vi "Tosca-Randomize Parameter Family.vi"(0 "Family in":T1, 7 "Mode":T5, 11 "N":i32) -> (4 "Family thru":T1, 8 "SCL":T6[](array[typedef]))   [LabVIEW 2020]
uses:
  Typedefs/Tosca-Parameter Family.ctl
  Typedefs/Tosca-Parameter Table Element.ctl
  Typedefs/Tosca-Parameter Dimension.ctl
  Typedefs/Tosca-Family Order.ctl
  Typedefs/Tosca-SCL Element.ctl
  Typedefs/Tosca-Schedule Mode.ctl
  Typedefs/Tosca-Event Type.ctl
  Typedefs/Tosca-SCL Variable.ctl
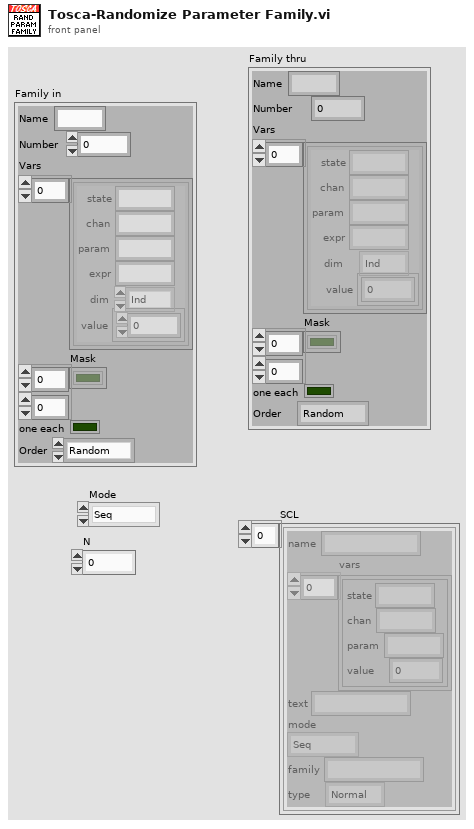
[diagram p1: front panel]
types:
  T1 = typedef "Tosca-Parameter Family.ctl" = cluster{"Name":string, "Number":i32, "Vars":T2[], "Mask":bool[][], "one each":bool, "Order":T4}
  T2 = typedef "Tosca-Parameter Table Element.ctl" = cluster{"state":string, "chan":string, "param":string, "expr":string, "dim":T3, "value":dbl[]}
  T3 = typedef "Tosca-Parameter Dimension.ctl" = enum16{"Ind", "X", "Y"}
  T4 = typedef "Tosca-Family Order.ctl" = enum16{"Random", "Sequential"}
  T5 = typedef "Tosca-Schedule Mode.ctl" = enum16{"Seq", "CS+/CS-", "Adapt"}
  T6 = typedef "Tosca-SCL Element.ctl" = cluster{"name":string, "vars":cluster{"state":string, "chan":string, "param":string, "value":dbl}[], "text":string, "mode":T5, "family":string, "type":T7}
  T7 = typedef "Tosca-Event Type.ctl" = enum16{"Normal", "CS+", "CS-"}
  T8 = typedef "Tosca-SCL Variable.ctl" = cluster{"state":string, "chan":string, "param":string, "value":dbl}
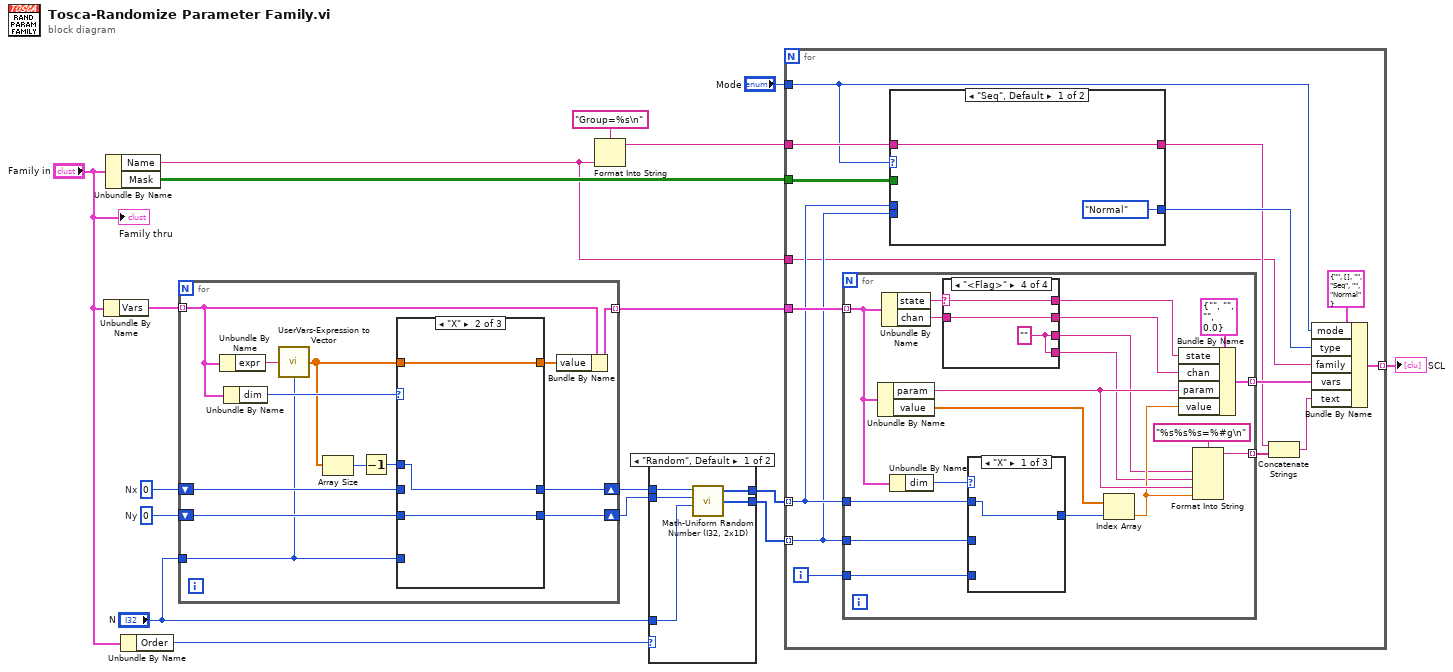
[diagram p0: block diagram]
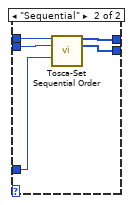
[diagram p2: hidden frame]
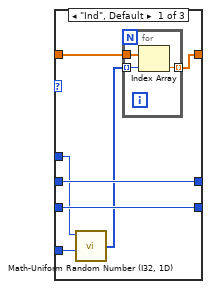
[diagram p3: hidden frame]
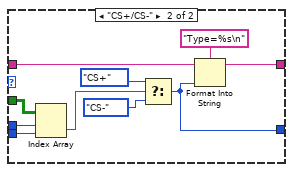
[diagram p5: hidden frame]
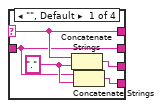
[diagram p6: hidden frame]
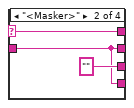
[diagram p7: hidden frame]
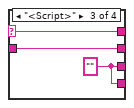
[diagram p8: hidden frame]
diagram:
  w15 = 0  # Ny
  w16 = 0  # Nx
  n1 = Unbundle By Name("Family in") -> ("Vars"=w17:T2[])
  n2 = Unbundle By Name("Family in") -> ("Name"=w8:string, "Mask"=w11:bool[][])
  n3 = Unbundle By Name("Family in") -> ("Order"=w1:T4)
  n4 = for {
    tunnel: w17 -> [w23] mode=indexing
    shift-right: [w27] -> w5
    shift-left: w16 -> [w26]
    shift-right: [w25] -> w4
    shift-left: w15 -> [w24]
    tunnel: [w22] -> w14 mode=indexing
    tunnel: "N" -> [w18]
    n5 = Unbundle By Name(w23) -> ("expr"=w30:string)
    n6 = Unbundle By Name(w23) -> ("dim"=w29:T3)
    n7 = call "UserVars-Expression to Vector.vi"("Expr"=w30, "Nrand"=w18) -> ("Values"=w20:dbl[])  [unwired: 12 in, 1 out]
    n8 = Array Size(array=w20) -> (size(s)=w28:i32)
    n9 = Decrement(x=w28) -> (x-1=w19:i32)
    n10 = case shown="\"X\"" w29 {
      tunnel: w19 -> [w35 w42 w46]
      tunnel: [w37 w42 w45] -> w27
      tunnel: w26 -> [w37 _ w45]
      tunnel: [w36 w43 w46] -> w25
      tunnel: w24 -> [w36 w43 _]
      tunnel: w18 -> [w34 _ _]
      tunnel: [w32 w41 w44] -> w21
      tunnel: w20 -> [w33 w41 w44]
      frame "Ind", Default {
        n11 = call "Math-Uniform Random Number (I32, 1D).vi"("N"=w34, "Ymax"=w35) -> ("Random Ints"=w31:i32[])  [unwired: 4 in]
        n12 = for {
          tunnel: w33 -> [w40]
          tunnel: [w39] -> w32 mode=indexing
          tunnel: w31 -> [w38] mode=indexing
          n13 = Index Array(array=w40, index=w38) -> (element=w39:dbl)
        }
      }
      frame "X" {
      }
      frame "Y" {
      }
    }
    n14 = Bundle By Name(cluster=w23, "value"=w21) -> (w22:T2)
  }
  n15 = Format Into String(format string="Group=%s\n", w8) -> (resulting string=w12:string)  [unwired: 2 in, 1 out]
  n16 = case shown="\"Random\", Default" w1 {
    tunnel: "N" -> [w51 w54]
    tunnel: [w50 w52] -> w6
    tunnel: w5 -> [w49 w56]
    tunnel: w4 -> [w48 w55]
    tunnel: [w47 w53] -> w3
    frame "Random", Default {
      n17 = call "Math-Uniform Random Number (I32, 2x1D).vi"("N"=w51, "Ymax"=w48, "Xmax"=w49) -> ("Yi"=w50:i32[], "Xi"=w47:i32[])  [unwired: 2 in]
    }
    frame "Sequential" {
      n18 = call "Tosca-Set Sequential Order.vi"("Nx"=w56, "Ny"=w55, "N"=w54) -> ("ix"=w53:i32[], "iy"=w52:i32[])  [unwired: 11 in]
    }
  }
  n19 = for {
    tunnel: w14 -> [w71]
    tunnel: w3 -> [w64] mode=indexing
    tunnel: w6 -> [w63] mode=indexing
    tunnel: w12 -> [w60]
    tunnel: w11 -> [w65]
    tunnel: [w61] -> w10 mode=indexing
    tunnel: "Mode" -> [w58]
    tunnel: w8 -> [w57]
    i -> [w70]
    n20 = for {
      tunnel: w71 -> [w90] mode=indexing
      tunnel: w70 -> [w99]
      tunnel: w64 -> [w97]
      tunnel: w63 -> [w96]
      tunnel: [w92] -> w67 mode=indexing
      tunnel: [w91] -> w68 mode=indexing
      n21 = Unbundle By Name(w90) -> ("param"=w98:string, "value"=w95:dbl[])
      n22 = Unbundle By Name(w90) -> ("state"=w89:string, "chan"=w87:string)
      n23 = Unbundle By Name(w90) -> ("dim"=w100:T3)
      n24 = case shown="\"<Flag>\"" w89 {
        selector: w89 -> [w104 w109 w112 w115]
        tunnel: [w107 "" w113 w116] -> w85
        tunnel: [w106 w108 w113 w116] -> w84
        tunnel: [w104 w109 w112 w115] -> w88
        tunnel: w87 -> [w103 w108 w111 w114]
        tunnel: [w103 w108 w111 w114] -> w86
        frame "", Default {
          w105 = "."
          n25 = Concatenate Strings(w104, w105) -> (w107:string)
          n26 = Concatenate Strings(w103, w105) -> (w106:string)
        }
        frame "<Masker>" {
        }
        frame "<Script>" {
          w113 = ""
        }
        frame "<Flag>" {
          w116 = ""
        }
      }
      n27 = case shown="\"X\"" w100 {
        tunnel: w99 -> [_ w118 _]
        tunnel: w97 -> [w117 _ _]
        tunnel: w96 -> [_ _ w119]
        tunnel: [w117 w118 w119] -> w93
        frame "X" {
        }
        frame "Ind", Default {
        }
        frame "Y" {
        }
      }
      n28 = Index Array(array=w95, index=w93) -> (element=w94:dbl)
      n29 = Bundle By Name(cluster=T8 {"state"="", "chan"="", "param"="", "value"=0.0} ("var"), "state"=w88, "chan"=w86, "param"=w98, "value"=w94) -> (w91:T8)
      n30 = Format Into String(format string="%s%s%s=%#g\n", w85, w84, w98, w94) -> (resulting string=w92:string)  [unwired: 2 in, 1 out]
    }
    n31 = case shown="\"Seq\", Default" w58 {
      tunnel: w65 -> [_ w83]
      tunnel: w64 -> [_ w82]
      tunnel: w63 -> [_ w81]
      tunnel: [Tosca-Event_Type."Normal" ("type") w74] -> w62
      tunnel: w60 -> [w73 w80]
      tunnel: [w73 w79] -> w59
      frame "Seq", Default {
      }
      frame "CS+/CS-" {
        n32 = Index Array(array=w83, index (row)=w82, index (col)=w81) -> (element=w77:bool)
        n33 = Select(t=Tosca-Event_Type."CS+" ("type"), s=w77, f=Tosca-Event_Type."CS-" ("type")) -> (s? t:f=w74:T7)
        n34 = Format Into String(format string="Type=%s\n", initial string=w80, w74) -> (resulting string=w79:string)  [unwired: 1 in, 1 out]
      }
    }
    n35 = Concatenate Strings(w59, w67) -> (w66:string)
    n36 = Bundle By Name(cluster=T6 {"name"="", "vars"=[], "text"="", "mode"=enum."Seq", "family"="", "type"=enum."Normal"} ("StimCon"), "mode"=w58, "type"=w62, "family"=w57, "vars"=w68, "text"=w66) -> (w61:T6)
  }
  "SCL" <- w10
  "Family thru" <- "Family in"
